vi "AutoDrive.vi"(9 "Initialized":bool) -> (2 "Drive State":T3=enum."Follow Path")   [LabVIEW 2018]
uses:
  driveStateEnum.ctl
  MotionProfile/Path_Decider.ctl
  MotionProfile/StartingPosition.ctl
  AutoDriveStates.ctl
  MotionProfile/AutoOptions.ctl
  Sensors/Limelight/LimelightPipelineMode.ctl
  <userlib>/836-Library/System/TDMS_V2/Support/TDMS_DevRef.ctl
  <userlib>/836-Library/System/TDMS_V2/Support/Logging_Settings.ctl
  <userlib>/836-Library/System/TDMS_V2/Support/Group_FIFO_Config.ctl
  <userlib>/836-Library/System/TDMS_V2/Support/Channel_FIFO_Config.ctl
  HatchPanel/hatchPanelEnum.ctl
  HatchPanel/hatchPanelNotifierCluster.ctl
  Sensors/Limelight/LimelightModeEnum.ctl
  driveShifterEnum.ctl
  MotionProfile/Constants.vi
panel:
  in  "Override Dashboard":bool
  out "Complete Path Valid?":bool
  in  "Starting Position":T1
  in  "Second":T2=enum."5"
  in  "First":T2=enum."7"
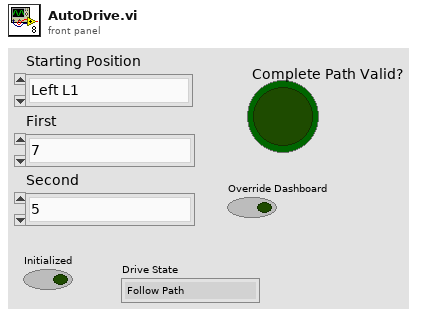
[diagram p1: front panel]
types:
  T1 = typedef "StartingPosition.ctl" = enum16{"Left L1 ", "Middle L1", "Right L1", "Left L2", "Right L2", "Don't Move"}
  T2 = typedef "Path_Decider.ctl" = enum16{"1", "2", "3", "4", "5", "6", "7", "8", "Left_Rocket_Front", "Left_Rocket_Rear", "Right_Rocket_Front", "Right_Rocket_Rear"}
  T3 = typedef "driveStateEnum.ctl" = enum16{"doNothing", "Manuel", "Teleop", "Follow Path (init)", "Follow Path", "Move to Target", "Climb", "Line Align", "Turn to Angle", "Sonar Brake Tele", "Code Drive"}
  T4 = typedef "AutoDriveStates.ctl" = enum16{"1 - MP First leg A (init)", "2 - MP First leg A", "3 - Wait for direction change", "4 - MP First leg B (init)", "5 - MP First leg B", "6 - Wait for shift", "7 - Aproach to score", "8 - Scored", "9 - MP Second leg A (init)", "10 - MP Second leg A", "11 - Wait for direction change", "12 - MP Second leg B (init)", "13 - MP Second leg B", "14 - Wait for shift", "15 - Extend claw", "16 - Aproach to grab", "17 - Grabbed", "18 - MP Third leg A (init)", "19 - MP Third leg A", "20 - Wait for direction change", "21 - MP Third leg B (init)", "22 - MP Third leg B", "23 - Wait to shift", "24 - Aproach to score", "25 - Scored", "26 - Backup 0.3 Seconds", "27 - doNothing"}
  T5 = typedef "AutoOptions.ctl" = cluster{"Starting Position":T1, "First Score Pos":T2, "Second Score Pos":T2}
  T6 = typedef "LimelightPipelineMode.ctl" = enum16{"Closest", "Leftmost", "Rightmost"}
  T7 = typedef "pathLeg.ctl" = cluster{"First Path":string, "Second Path Needed?":bool, "Second Path":string}
  T8 = typedef "WPI_MotorControlDeviceRef.ctl" = cluster{"DeviceStatus":errorcluster, "Type":T9, "PWM":cluster{"PWM Channel":T10, "DeadBand":T11}, "CAN":cluster{"Device Number":u8, "SetOutput VI Ref":variant, "GetOutput VI Ref":variant, "Enable VI Ref":variant, "Disable VI Ref":variant, "Data":variant}, "Invert":bool, "DIO PWM":cluster{"PWM \"Enable\" Channel":T10, "DIOChannel":T12, "PWM Rate":dbl}}
  T9 = typedef "WPI_MotorControlType.ctl" = enum16{"PWM", "CAN", "DIO PWM"}
  T10 = typedef "FPGA_DIOPWMChannel.ctl" = enum8{"PWM 0", "PWM 1", "PWM 2", "PWM 3", "PWM 4", "PWM 5", "PWM 6", "PWM 7", "PWM 8", "PWM 9", "PWM MXP 0", "PWM MXP 1", "PWM MXP 2", "PWM MXP 3", "PWM MXP 4", "PWM MXP 5", "PWM MXP 6", "PWM MXP 7", "PWM MXP 8", "PWM MXP 9", "Invalid"}
  T11 = typedef "WPI_PWMDeadband.ctl" = cluster{"Name":string, "maxPositivePwm":i32, "minPositivePwm":i32, "centerPwm":i32, "maxNegativePwm":i32, "minNegativePwm":i32, "angularRange":u16}
  T12 = typedef "FPGA_DIOChannel.ctl" = enum8{"DIO 0", "DIO 1", "DIO 2", "DIO 3", "DIO 4", "DIO 5", "DIO 6", "DIO 7", "DIO 8", "DIO 9", "DIO MXP 0", "DIO MXP 1", "DIO MXP 2", "DIO MXP 3", "DIO MXP 4", "DIO MXP 5", "DIO MXP 6", "DIO MXP 7", "DIO MXP 8", "DIO MXP 9", "DIO MXP 10", "DIO MXP 11", "DIO MXP 12", "DIO MXP 13", "DIO MXP 14", "DIO MXP 15", "SPI Port CS1", "SPI Port CS2", "SPI Port CS3", "SPI Port MISO", "SPI Port MOSI", "Invalid"}
  T13 = typedef "driveShifterEnum.ctl" = enum16{"Low", "High"}
  T14 = typedef "LimelightModeEnum.ctl" = enum16{"SA - Front", "SA - Rear", "SA - Side by Side", "Vision Processing"}
  T15 = typedef "hatchPanelNotifierCluster.ctl" = cluster{"Hatch Panel State":T16, "Mechanism Motion":bool, "Gathering Claw Motion":bool, "Scoring Claw Motion":bool}
  T16 = typedef "hatchPanelEnum.ctl" = enum16{"do nothing", "Stach Mode", "Climb Mode", "Retracted Closed", "Retracted Open", "Extended Closed", "Extended Open"}
  T17 = typedef "CTRE_PigeonIMU_DeviceRef.ctl" = cluster{"DeviceStatus":errorcluster, "Device Number":u8, "Type":T18, "Device ID":u32, "Handle":u64, "UsageFrame":u32, "Library Path":path}
  T18 = typedef "CTRE_PigeonIMU_ConnectionType.ctl" = u32
  T19 = typedef "TDMS_DevRef.ctl" = cluster{"Name":string, "File Ref":refnum<k34>, "Start Time":timestamp, "Logging Settings":T20, "Group FIFO Config":T21[], "Data To Write":refnum<data-value>, "semaphore":T23, "Ref Time Reset":refnum<k4>}
  T20 = typedef "Logging_Settings.ctl" = cluster{"Data Grab Period":dbl, "File Write Period":dbl, "Max Stored Size":dbl, "Burst Size":dbl}
  T21 = typedef "Group_FIFO_Config.ctl" = cluster{"Group":string, "Channels":T22[], "Channel Names":string[]}
  T22 = typedef "Channel_FIFO_Config.ctl" = cluster{"Channel":string, "FIFO":refnum<k33>}
  T23 = typedef "Semaphore RefNum" = refnum<k1>
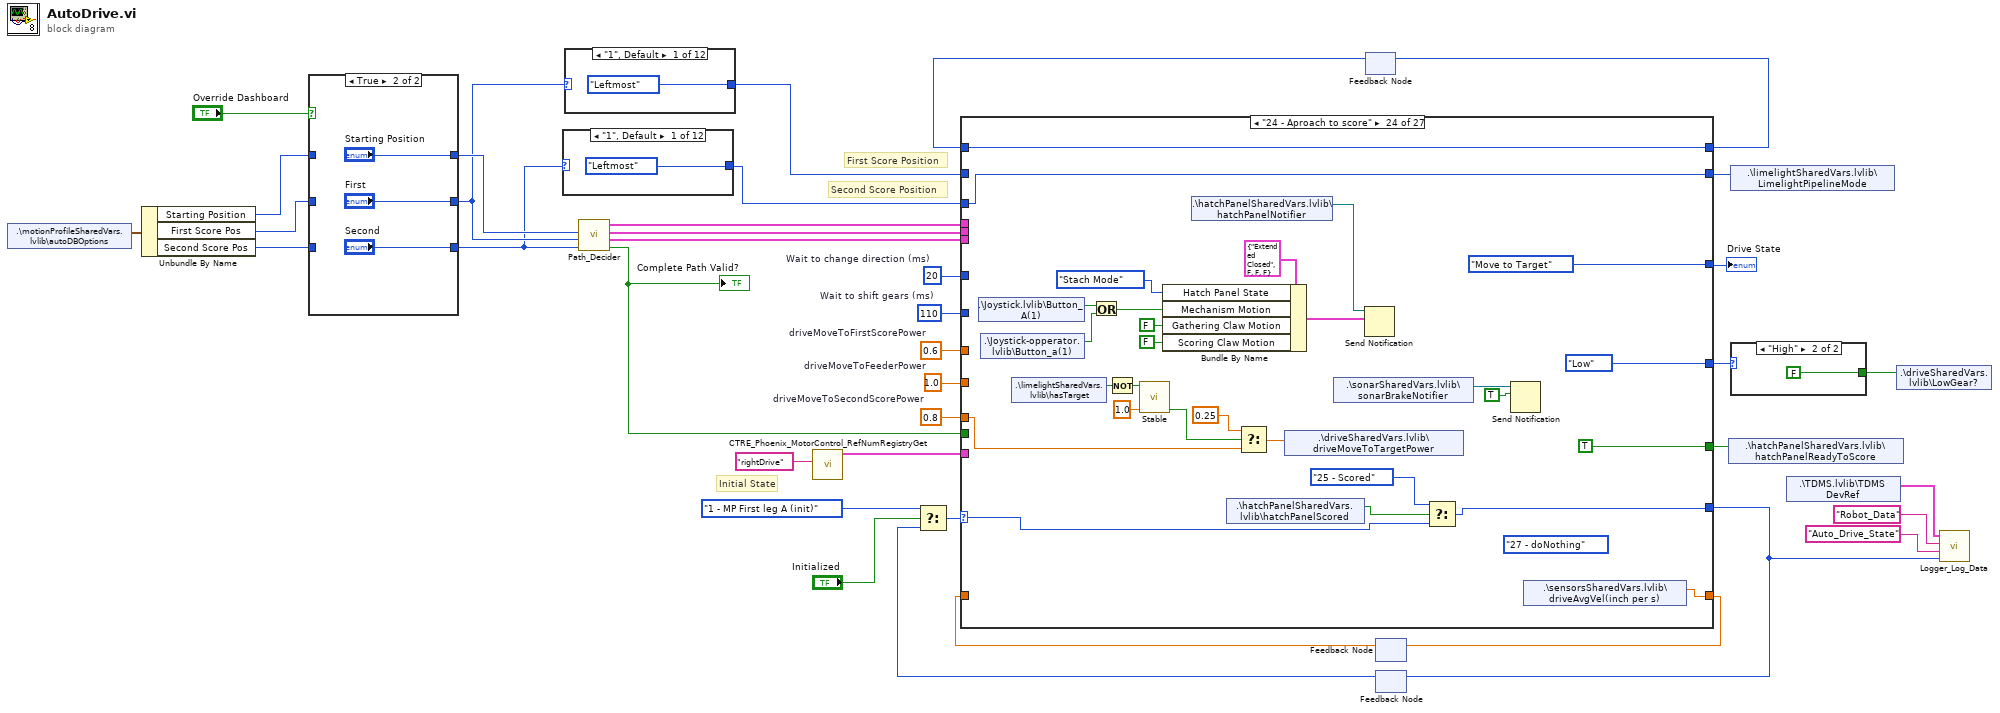
[diagram p0: block diagram]
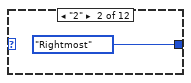
[diagram p2: hidden frame]
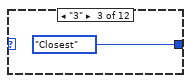
[diagram p3: hidden frame]
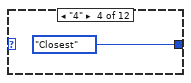
[diagram p4: hidden frame]
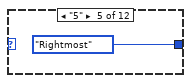
[diagram p5: hidden frame]
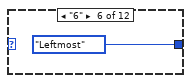
[diagram p6: hidden frame]
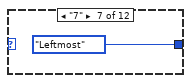
[diagram p7: hidden frame]
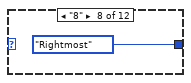
[diagram p8: hidden frame]
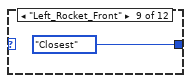
[diagram p9: hidden frame]
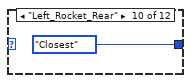
[diagram p10: hidden frame]
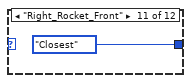
[diagram p11: hidden frame]
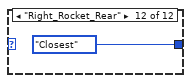
[diagram p12: hidden frame]
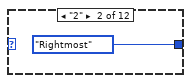
[diagram p13: hidden frame]
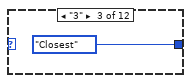
[diagram p14: hidden frame]
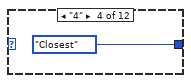
[diagram p15: hidden frame]
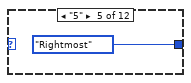
[diagram p16: hidden frame]
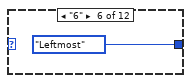
[diagram p17: hidden frame]
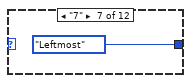
[diagram p18: hidden frame]
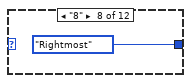
[diagram p19: hidden frame]
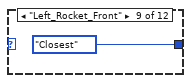
[diagram p20: hidden frame]
diagram:
  w9 = 0.8  # driveMoveToSecondScorePower
  w10 = 1.0  # driveMoveToFeederPower
  w23 = 0.6  # driveMoveToFirstScorePower
  w24 = u32 110  # Wait to shift gears (ms)
  w25 = u32 20  # Wait to change direction (ms)
  # "Second Score Position"
  # "First Score Position"
  # "Initial State"
  n1 = shared-variable ".\\motionProfileSharedVars.lvlib\\autoDBOptions"() -> (w17:T5)  [unwired: 1 in, 1 out]
  n2 = Unbundle By Name(w17) -> ("Starting Position"=w19:T1, "First Score Pos"=w20:T2, "Second Score Pos"=w21:T2)
  n3 = case shown="True" "Override Dashboard" {
    tunnel: [w40 "First"] -> w5
    tunnel: [w41 "Second"] -> w2
    tunnel: [w39 "Starting Position"] -> w6
    tunnel: w21 -> [w41 _]
    tunnel: w20 -> [w40 _]
    tunnel: w19 -> [w39 _]
    frame False {
    }
    frame True {
    }
  }
  n4 = case shown="\"1\", Default" w2 {
    tunnel: [LimelightPipelineMode."Leftmost" ("Enum") LimelightPipelineMode."Rightmost" ("Enum") LimelightPipelineMode."Closest" ("Enum") LimelightPipelineMode."Closest" ("Enum") LimelightPipelineMode."Rightmost" ("Enum") LimelightPipelineMode."Leftmost" ("Enum") LimelightPipelineMode."Leftmost" ("Enum") LimelightPipelineMode."Rightmost" ("Enum") LimelightPipelineMode."Closest" ("Enum") LimelightPipelineMode."Closest" ("Enum") LimelightPipelineMode."Closest" ("Enum") LimelightPipelineMode."Closest" ("Enum")] -> w1
    frame "1", Default {
    }
    frame "2" {
    }
    frame "3" {
    }
    frame "4" {
    }
    frame "5" {
    }
    frame "6" {
    }
    frame "7" {
    }
    frame "8" {
    }
    frame "Left_Rocket_Front" {
    }
    frame "Left_Rocket_Rear" {
    }
    frame "Right_Rocket_Front" {
    }
    frame "Right_Rocket_Rear" {
    }
  }
  n5 = case shown="\"1\", Default" w5 {
    tunnel: [LimelightPipelineMode."Leftmost" ("Enum") LimelightPipelineMode."Rightmost" ("Enum") LimelightPipelineMode."Closest" ("Enum") LimelightPipelineMode."Closest" ("Enum") LimelightPipelineMode."Rightmost" ("Enum") LimelightPipelineMode."Leftmost" ("Enum") LimelightPipelineMode."Leftmost" ("Enum") LimelightPipelineMode."Rightmost" ("Enum") LimelightPipelineMode."Closest" ("Enum") LimelightPipelineMode."Closest" ("Enum") LimelightPipelineMode."Closest" ("Enum") LimelightPipelineMode."Closest" ("Enum")] -> w4
    frame "1", Default {
    }
    frame "2" {
    }
    frame "3" {
    }
    frame "4" {
    }
    frame "5" {
    }
    frame "6" {
    }
    frame "7" {
    }
    frame "8" {
    }
    frame "Left_Rocket_Front" {
    }
    frame "Left_Rocket_Rear" {
    }
    frame "Right_Rocket_Front" {
    }
    frame "Right_Rocket_Rear" {
    }
  }
  n6 = call "Path_Decider.vi"("Second"=w2, "First"=w5, "Starting Position"=w6) -> ("Complete Path Valid?"=w18:bool, "Score Second HP Leg"=w26:T7, "Retrieve Second HP Leg"=w27:T7, "Score First HP Leg"=w28:T7)  [unwired: 4 in]
  "Complete Path Valid?" <- w18
  n7 = call <vilib>:"CTRE_Phoenix_MotorControl_RefNumRegistryGet.vi"("refnum name"="rightDrive") -> ("PhoenixMotorControlDevRef"=w37:T8)  [unwired: 9 in, 1 out]
  n8 = feedback #1() -> (w33:u32)  [unwired: 1 in]
  n9 = feedback #2() -> (w7:dbl)  [unwired: 1 in]
  n10 = feedback #3() -> (w29:T4)  [unwired: 1 in]
  n11 = Select(t=AutoDriveStates."1 - MP First leg A (init)" ("Enum"), s="Initialized", f=w29) -> (s? t:f=w30:T4)
  n12 = case shown="\"24 - Aproach to score\"" w30 {
    selector: w30 -> [_ w122 w139 _ w175 w184 w217 _ _ w272 w293 _ w333 w341 _ w376 _ _ w450 w471 _ w507 w516 w548 _ w576 _]
    tunnel: [w86 w101 w124 AutoDriveStates."5 - MP First leg B" ("Enum") w177 w183 w194 AutoDriveStates."9 - MP Second leg A (init)" ("Enum") AutoDriveStates."10 - MP Second leg A" ("Enum") w271 w278 AutoDriveStates."13 - MP Second leg B" ("Enum") w320 w335 AutoDriveStates."16 - Aproach to grab" ("t") w355 AutoDriveStates."18 - MP Third leg A (init)" ("Enum") AutoDriveStates."19 - MP Third leg A" ("Enum") w449 w456 AutoDriveStates."22 - MP Third leg B" ("Enum") w506 w515 w526 AutoDriveStates."26 - Backup 0.3 Seconds" ("Enum") w575 AutoDriveStates."27 - doNothing" ("Enum")] -> w11
    tunnel: [driveStateEnum."Follow Path (init)" ("Drive State Enum") driveStateEnum."Follow Path" ("Drive State Enum") driveStateEnum."doNothing" ("Drive State Enum") driveStateEnum."Follow Path (init)" ("Drive State Enum") driveStateEnum."Follow Path" ("Drive State Enum") driveStateEnum."doNothing" ("Drive State Enum") driveStateEnum."Move to Target" ("Drive State Enum") driveStateEnum."doNothing" ("Drive State Enum") driveStateEnum."Follow Path (init)" ("Drive State Enum") driveStateEnum."Follow Path" ("Drive State Enum") driveStateEnum."doNothing" ("Drive State Enum") driveStateEnum."Follow Path (init)" ("Drive State Enum") driveStateEnum."Follow Path" ("Drive State Enum") driveStateEnum."doNothing" ("Drive State Enum") driveStateEnum."doNothing" ("Drive State Enum") driveStateEnum."Move to Target" ("Drive State Enum") driveStateEnum."doNothing" ("Drive State Enum") driveStateEnum."Follow Path (init)" ("Drive State Enum") driveStateEnum."Follow Path" ("Drive State Enum") driveStateEnum."doNothing" ("Drive State Enum") driveStateEnum."Follow Path (init)" ("Drive State Enum") driveStateEnum."Follow Path" ("Drive State Enum") driveStateEnum."doNothing" ("Drive State Enum") driveStateEnum."Move to Target" ("Drive State Enum") driveStateEnum."doNothing" ("Drive State Enum") driveStateEnum."Code Drive" ("Drive State Enum") driveStateEnum."doNothing" ("Drive State Enum")] -> w35
    tunnel: w37 -> [_ w121 _ _ w176 _ _ _ _ w273 _ _ w332 _ _ _ _ _ w451 _ _ w508 _ _ _ _ _]
    tunnel: [w73 w109 w130 w148 w167 driveShifterEnum."Low" ("driveShifterPosition") driveShifterEnum."Low" ("driveShifterPosition") driveShifterEnum."Low" ("driveShifterPosition") w242 w261 w284 w302 w322 driveShifterEnum."Low" ("driveShifterPosition") driveShifterEnum."Low" ("driveShifterPosition") driveShifterEnum."Low" ("driveShifterPosition") driveShifterEnum."High" ("driveShifterPosition") w401 w439 w462 w480 w499 driveShifterEnum."Low" ("driveShifterPosition") driveShifterEnum."Low" ("driveShifterPosition") driveShifterEnum."Low" ("driveShifterPosition") driveShifterEnum."Low" ("driveShifterPosition") driveShifterEnum."High" ("driveShifterPosition")] -> w16
    tunnel: [w97 w119 w143 w157 w173 w186 w220 w235 w253 w274 w297 w311 w330 w345 w352 w378 w393 w418 w452 w475 w489 w509 w518 w551 w563 w577 w588] -> w34
    tunnel: w33 -> [w97 _ w143 w157 _ w186 w220 w235 w253 _ w297 w311 _ w345 w352 w378 w393 w418 _ w475 w489 _ w518 w551 _ w577 w588]
    tunnel: [FALSE FALSE FALSE FALSE FALSE FALSE TRUE FALSE FALSE FALSE FALSE FALSE FALSE FALSE TRUE TRUE FALSE FALSE FALSE FALSE FALSE FALSE FALSE TRUE FALSE FALSE FALSE] -> w32
    tunnel: w28 -> [w87 w117 w128 w155 w174 _ _ _ _ _ _ _ _ _ _ _ _ _ _ _ _ _ _ _ _ _ _]
    tunnel: w27 -> [_ _ _ _ _ _ _ _ w249 w270 w282 w309 w328 _ _ _ _ _ _ _ _ _ _ _ _ _ _]
    tunnel: w26 -> [_ _ _ _ _ _ _ _ _ _ _ _ _ _ _ _ _ w416 w445 w460 w487 w505 _ _ _ _ _]
    tunnel: w25 -> [_ _ w137 _ _ _ _ _ _ _ w291 _ _ _ _ _ _ _ _ w469 _ _ _ _ _ _ _]
    tunnel: w24 -> [_ _ _ _ _ w185 _ _ _ _ _ _ _ w338 _ _ _ _ _ _ _ _ w517 _ _ _ _]
    tunnel: w23 -> [_ _ _ _ _ _ _ _ _ _ _ _ _ _ _ _ _ _ _ _ _ _ _ _ _ _ _]
    tunnel: w18 -> [w84 _ _ _ _ _ _ _ _ _ _ _ _ _ _ _ _ _ _ _ _ _ _ _ _ _ _]
    tunnel: w10 -> [_ _ _ _ _ _ _ _ _ _ _ _ _ _ _ w365 _ _ _ _ _ _ _ _ _ _ _]
    tunnel: w9 -> [_ _ _ _ _ _ _ _ _ _ _ _ _ _ _ _ _ _ _ _ _ _ _ w538 _ _ _]
    tunnel: [w70 w102 w127 w146 w161 w182 w204 w231 w240 w255 w281 w300 w315 w337 w349 w364 w389 w399 w433 w459 w478 w493 w514 w537 w562 w571 w586] -> w8
    tunnel: w7 -> [_ _ _ _ _ _ w204 _ _ _ _ _ _ _ _ _ _ _ _ _ _ _ _ _ _ _ w586]
    tunnel: w4 -> [w69 w100 w126 w145 w160 w181 w202 w230 _ _ _ _ _ _ _ _ _ _ _ _ _ _ _ _ _ _ _]
    tunnel: w1 -> [_ _ _ _ _ _ _ _ _ _ _ _ _ _ _ _ _ w398 w432 w458 w477 w492 w513 w536 w561 w570 w585]
    tunnel: [w69 w100 w126 w145 w160 w181 w202 w230 LimelightPipelineMode."Closest" ("Enum") LimelightPipelineMode."Closest" ("Enum") LimelightPipelineMode."Closest" ("Enum") LimelightPipelineMode."Closest" ("Enum") LimelightPipelineMode."Closest" ("Enum") LimelightPipelineMode."Closest" ("Enum") LimelightPipelineMode."Closest" ("Enum") LimelightPipelineMode."Closest" ("Enum") LimelightPipelineMode."Closest" ("Enum") w398 w432 w458 w477 w492 w513 w536 w561 w570 w585] -> w3
    frame "1 - MP First leg A (init)", Default {
      n13 = shared-variable ".\\limelightSharedVars.lvlib\\limelightModeNotifier"() -> (w82:refnum<notifier>)  [unwired: 1 in, 1 out]
      n14 = shared-variable ".\\sonarSharedVars.lvlib\\sonarBrakeNotifier"() -> (w72:refnum<notifier>)  [unwired: 1 in, 1 out]
      n15 = Unbundle By Name(w87) -> ("First Path"=w74:string)
      n16 = call <vilib>:"CTRE_PigeonIMU_RefNumRegistryGet.vi"("refnum name"="driveIMU") -> ("PigeonIMUDevRef"=w88:T17)  [unwired: 9 in, 1 out]
      n17 = call "ZeroPigeon.vi"("Pigeon"=w88) -> ()  [unwired: 8 in, 1 out]
      n18 = shared-variable ".\\motionProfileSharedVars.lvlib\\motionProfilePathName"(w74) -> ()  [unwired: 1 in, 1 out]
      n19 = Send Notification(notification=LimelightModeEnum."Vision Processing", notifier=w82) -> ()  [unwired: 1 in, 2 out]
      n20 = Send Notification(notification=FALSE, notifier=w72) -> ()  [unwired: 1 in, 2 out]
      n21 = Bundle By Name(cluster=T15 {"Hatch Panel State"=enum."Extended Closed", "Mechanism Motion"=FALSE, "Gathering Claw Motion"=FALSE, "Scoring Claw Motion"=FALSE} ("notification"), "Hatch Panel State"=hatchPanelEnum."Stach Mode", "Mechanism Motion"=FALSE, "Gathering Claw Motion"=FALSE, "Scoring Claw Motion"=FALSE) -> (w94:T15)
      n22 = String Subset(string=w74, length (rest)=4 ("length (rest)")) -> (substring=w79:string)  [unwired: 1 in]
      n23 = shared-variable ".\\hatchPanelSharedVars.lvlib\\hatchPanelNotifier"() -> (w95:refnum<notifier>)  [unwired: 1 in, 1 out]
      n24 = Equal?(x="low_", y=w79) -> (x = y?=w75:bool)
      n25 = Send Notification(notification=w94, notifier=w95) -> ()  [unwired: 1 in, 2 out]
      n26 = shared-variable ".\\sensorsSharedVars.lvlib\\driveAvgVel(inch per s)"() -> (w70:dbl)  [unwired: 1 in, 1 out]
      n27 = Select(t=driveShifterEnum."Low" ("driveShifterPosition"), s=w75, f=driveShifterEnum."High" ("driveShifterPosition")) -> (s? t:f=w73:T13)
      n28 = Select(t=AutoDriveStates."2 - MP First leg A" ("Enum"), s=w84, f=AutoDriveStates."27 - doNothing" ("Enum")) -> (s? t:f=w86:T4)
    }
    frame "2 - MP First leg A" {
      n29 = call <vilib>:"CTRE_Phoenix_MotorControl_IsMotionProfileFinished.vi"("PhoenixMotorControlDevRef"=w121) -> ("Is Motion Profile Finished?"=w120:bool)  [unwired: 8 in, 2 out]
      n30 = Unbundle By Name(w117) -> ("First Path"=w110:string, "Second Path Needed?"=w114:bool)
      n31 = shared-variable ".\\motionProfileSharedVars.lvlib\\motionProfilePathName"(w110) -> ()  [unwired: 1 in, 1 out]
      n32 = String Subset(string=w110, length (rest)=4 ("length (rest)")) -> (substring=w112:string)  [unwired: 1 in]
      n33 = Equal?(x="low_", y=w112) -> (x = y?=w105:bool)
      n34 = shared-variable ".\\sensorsSharedVars.lvlib\\driveAvgVel(inch per s)"() -> (w102:dbl)  [unwired: 1 in, 1 out]
      n35 = Select(t=AutoDriveStates."7 - Aproach to score", s=w105, f=AutoDriveStates."6 - Wait for shift" ("t")) -> (s? t:f=w106:T4)
      n36 = Select(t=AutoDriveStates."3 - Wait for direction change", s=w114, f=w106) -> (s? t:f=w116:T4)
      n37 = Select(t=w116, s=w120, f=w122) -> (s? t:f=w101:T4)
      n38 = Tick Count (ms)() -> (millisecond timer value=w119:u32)
      n39 = Select(t=driveShifterEnum."Low" ("driveShifterPosition"), s=w105, f=driveShifterEnum."High" ("driveShifterPosition")) -> (s? t:f=w109:T13)
    }
    frame "3 - Wait for direction change" {
      n40 = Add(x=w143, y=w137) -> (x+y=w141:u32)
      n41 = Unbundle By Name(w128) -> ("Second Path"=w129:string)
      n42 = Tick Count (ms)() -> (millisecond timer value=w142:u32)
      n43 = Greater Or Equal?(x=w142, y=w141) -> (x >= y?=w140:bool)
      n44 = String Subset(string=w129, length (rest)=4 ("length (rest)")) -> (substring=w135:string)  [unwired: 1 in]
      n45 = Equal?(x="low_", y=w135) -> (x = y?=w131:bool)
      n46 = shared-variable ".\\sensorsSharedVars.lvlib\\driveAvgVel(inch per s)"() -> (w127:dbl)  [unwired: 1 in, 1 out]
      n47 = Select(t=AutoDriveStates."4 - MP First leg B (init)", s=w140, f=w139) -> (s? t:f=w124:T4)
      n48 = Select(t=driveShifterEnum."Low" ("driveShifterPosition"), s=w131, f=driveShifterEnum."High" ("driveShifterPosition")) -> (s? t:f=w130:T13)
    }
    frame "4 - MP First leg B (init)" {
      n49 = Unbundle By Name(w155) -> ("Second Path"=w147:string)
      n50 = shared-variable ".\\motionProfileSharedVars.lvlib\\motionProfilePathName"(w147) -> ()  [unwired: 1 in, 1 out]
      n51 = String Subset(string=w147, length (rest)=4 ("length (rest)")) -> (substring=w153:string)  [unwired: 1 in]
      n52 = Equal?(x="low_", y=w153) -> (x = y?=w149:bool)
      n53 = shared-variable ".\\sensorsSharedVars.lvlib\\driveAvgVel(inch per s)"() -> (w146:dbl)  [unwired: 1 in, 1 out]
      n54 = Select(t=driveShifterEnum."Low" ("driveShifterPosition"), s=w149, f=driveShifterEnum."High" ("driveShifterPosition")) -> (s? t:f=w148:T13)
    }
    frame "5 - MP First leg B" {
      n55 = Unbundle By Name(w174) -> ("Second Path"=w166:string)
      n56 = call <vilib>:"CTRE_Phoenix_MotorControl_IsMotionProfileFinished.vi"("PhoenixMotorControlDevRef"=w176) -> ("Is Motion Profile Finished?"=w178:bool)  [unwired: 8 in, 2 out]
      n57 = shared-variable ".\\motionProfileSharedVars.lvlib\\motionProfilePathName"(w166) -> ()  [unwired: 1 in, 1 out]
      n58 = String Subset(string=w166, length (rest)=4 ("length (rest)")) -> (substring=w171:string)  [unwired: 1 in]
      n59 = Equal?(x="low_", y=w171) -> (x = y?=w162:bool)
      n60 = Select(t=AutoDriveStates."7 - Aproach to score" ("Enum"), s=w162, f=AutoDriveStates."6 - Wait for shift" ("Enum")) -> (s? t:f=w164:T4)
      n61 = shared-variable ".\\sensorsSharedVars.lvlib\\driveAvgVel(inch per s)"() -> (w161:dbl)  [unwired: 1 in, 1 out]
      n62 = Select(t=w164, s=w178, f=w175) -> (s? t:f=w177:T4)
      n63 = Tick Count (ms)() -> (millisecond timer value=w173:u32)
      n64 = Select(t=driveShifterEnum."Low" ("driveShifterPosition"), s=w162, f=driveShifterEnum."High" ("driveShifterPosition")) -> (s? t:f=w167:T13)
    }
    frame "6 - Wait for shift" {
      n65 = Add(x=w186, y=w185) -> (x+y=w189:u32)
      n66 = Tick Count (ms)() -> (millisecond timer value=w190:u32)
      n67 = Greater Or Equal?(x=w190, y=w189) -> (x >= y?=w188:bool)
      n68 = shared-variable ".\\sensorsSharedVars.lvlib\\driveAvgVel(inch per s)"() -> (w182:dbl)  [unwired: 1 in, 1 out]
      n69 = Select(t=AutoDriveStates."7 - Aproach to score", s=w188, f=w184) -> (s? t:f=w183:T4)
    }
    frame "7 - Aproach to score" {
      (unwired) AutoDriveStates."27 - doNothing" ("t")
      w207 = 100.0  # MaxLowGearSpeed (in/s)
      # "8.34457 ft/s Max Low Gear Speed"
      n70 = shared-variable ".\\limelightSharedVars.lvlib\\hasTarget"() -> (w213:bool)  [unwired: 1 in, 1 out]
      n71 = Not(x=w213) -> (.not. x?=w212:bool)
      n72 = Bundle By Name(cluster=T15 {"Hatch Panel State"=enum."Extended Closed", "Mechanism Motion"=FALSE, "Gathering Claw Motion"=FALSE, "Scoring Claw Motion"=FALSE} ("notification"), "Hatch Panel State"=hatchPanelEnum."Stach Mode", "Mechanism Motion"=TRUE, "Gathering Claw Motion"=FALSE, "Scoring Claw Motion"=FALSE) -> (w200:T15)
      n73 = Divide(x=w204, y=w207) -> (x/y=w206:dbl)
      n74 = shared-variable ".\\hatchPanelSharedVars.lvlib\\hatchPanelNotifier"() -> (w201:refnum<notifier>)  [unwired: 1 in, 1 out]
      n75 = call <userlib>:"Stable.vi"("Eval Period (sec)"=0.5, "Signal Input"=w212) -> ("Stable"=w210:bool)  [unwired: 9 in]
      n76 = Divide(x=w206, y=0.64) -> (x/y=w203:dbl)
      n77 = Select(t=0.25, s=w210, f=w203) -> (s? t:f=w208:dbl)
      n78 = shared-variable ".\\driveSharedVars.lvlib\\driveMoveToTargetPower"(w208) -> ()  [unwired: 1 in, 1 out]
      n79 = Send Notification(notification=w200, notifier=w201) -> ()  [unwired: 1 in, 2 out]
      n80 = shared-variable ".\\hatchPanelSharedVars.lvlib\\hatchPanelScored"() -> (w218:bool)  [unwired: 1 in, 1 out]
      n81 = shared-variable ".\\sonarSharedVars.lvlib\\sonarBrakeNotifier"() -> (w216:refnum<notifier>)  [unwired: 1 in, 1 out]
      n82 = Select(t=AutoDriveStates."8 - Scored", s=w218, f=w217) -> (s? t:f=w194:T4)
      n83 = Send Notification(notification=TRUE, notifier=w216) -> ()  [unwired: 1 in, 2 out]
    }
    frame "8 - Scored" {
      n84 = Bundle By Name(cluster=T15 {"Hatch Panel State"=enum."Extended Closed", "Mechanism Motion"=FALSE, "Gathering Claw Motion"=FALSE, "Scoring Claw Motion"=FALSE} ("notification"), "Hatch Panel State"=hatchPanelEnum."Stach Mode", "Mechanism Motion"=FALSE, "Gathering Claw Motion"=FALSE, "Scoring Claw Motion"=FALSE) -> (w228:T15)
      n85 = shared-variable ".\\hatchPanelSharedVars.lvlib\\hatchPanelNotifier"() -> (w229:refnum<notifier>)  [unwired: 1 in, 1 out]
      n86 = shared-variable ".\\sonarSharedVars.lvlib\\sonarBrakeNotifier"() -> (w234:refnum<notifier>)  [unwired: 1 in, 1 out]
      n87 = Send Notification(notification=w228, notifier=w229) -> ()  [unwired: 1 in, 2 out]
      n88 = Send Notification(notification=FALSE, notifier=w234) -> ()  [unwired: 1 in, 2 out]
      n89 = shared-variable ".\\sensorsSharedVars.lvlib\\driveAvgVel(inch per s)"() -> (w231:dbl)  [unwired: 1 in, 1 out]
    }
    frame "9 - MP Second leg A (init)" {
      n90 = Unbundle By Name(w249) -> ("First Path"=w241:string)
      n91 = shared-variable ".\\motionProfileSharedVars.lvlib\\motionProfilePathName"(w241) -> ()  [unwired: 1 in, 1 out]
      n92 = String Subset(string=w241, length (rest)=4 ("length (rest)")) -> (substring=w247:string)  [unwired: 1 in]
      n93 = Equal?(x="low_", y=w247) -> (x = y?=w243:bool)
      n94 = shared-variable ".\\sensorsSharedVars.lvlib\\driveAvgVel(inch per s)"() -> (w240:dbl)  [unwired: 1 in, 1 out]
      n95 = Select(t=driveShifterEnum."Low" ("driveShifterPosition"), s=w243, f=driveShifterEnum."High" ("driveShifterPosition")) -> (s? t:f=w242:T13)
    }
    frame "10 - MP Second leg A" {
      n96 = call <vilib>:"CTRE_Phoenix_MotorControl_IsMotionProfileFinished.vi"("PhoenixMotorControlDevRef"=w273) -> ("Is Motion Profile Finished?"=w275:bool)  [unwired: 8 in, 2 out]
      n97 = Unbundle By Name(w270) -> ("First Path"=w260:string, "Second Path Needed?"=w267:bool)
      n98 = shared-variable ".\\motionProfileSharedVars.lvlib\\motionProfilePathName"(w260) -> ()  [unwired: 1 in, 1 out]
      n99 = String Subset(string=w260, length (rest)=4 ("length (rest)")) -> (substring=w265:string)  [unwired: 1 in]
      n100 = Equal?(x="low_", y=w265) -> (x = y?=w258:bool)
      n101 = Select(t=AutoDriveStates."16 - Aproach to grab", s=w258, f=AutoDriveStates."14 - Wait for shift" ("t")) -> (s? t:f=w257:T4)
      n102 = shared-variable ".\\sensorsSharedVars.lvlib\\driveAvgVel(inch per s)"() -> (w255:dbl)  [unwired: 1 in, 1 out]
      n103 = Select(t=AutoDriveStates."11 - Wait for direction change", s=w267, f=w257) -> (s? t:f=w269:T4)
      n104 = Select(t=w269, s=w275, f=w272) -> (s? t:f=w271:T4)
      n105 = Tick Count (ms)() -> (millisecond timer value=w274:u32)
      n106 = Select(t=driveShifterEnum."Low" ("driveShifterPosition"), s=w258, f=driveShifterEnum."High" ("driveShifterPosition")) -> (s? t:f=w261:T13)
    }
    frame "11 - Wait for direction change" {
      (unwired) AutoDriveStates."27 - doNothing" ("t")
      n107 = Add(x=w297, y=w291) -> (x+y=w295:u32)
      n108 = Unbundle By Name(w282) -> ("Second Path"=w283:string)
      n109 = Tick Count (ms)() -> (millisecond timer value=w296:u32)
      n110 = Greater Or Equal?(x=w296, y=w295) -> (x >= y?=w294:bool)
      n111 = String Subset(string=w283, length (rest)=4 ("length (rest)")) -> (substring=w289:string)  [unwired: 1 in]
      n112 = Equal?(x="low_", y=w289) -> (x = y?=w285:bool)
      n113 = shared-variable ".\\sensorsSharedVars.lvlib\\driveAvgVel(inch per s)"() -> (w281:dbl)  [unwired: 1 in, 1 out]
      n114 = Select(t=AutoDriveStates."12 - MP Second leg B (init)", s=w294, f=w293) -> (s? t:f=w278:T4)
      n115 = Select(t=driveShifterEnum."Low" ("driveShifterPosition"), s=w285, f=driveShifterEnum."High" ("driveShifterPosition")) -> (s? t:f=w284:T13)
    }
    frame "12 - MP Second leg B (init)" {
      n116 = Unbundle By Name(w309) -> ("Second Path"=w301:string)
      n117 = shared-variable ".\\motionProfileSharedVars.lvlib\\motionProfilePathName"(w301) -> ()  [unwired: 1 in, 1 out]
      n118 = String Subset(string=w301, length (rest)=4 ("length (rest)")) -> (substring=w307:string)  [unwired: 1 in]
      n119 = Equal?(x="low_", y=w307) -> (x = y?=w303:bool)
      n120 = shared-variable ".\\sensorsSharedVars.lvlib\\driveAvgVel(inch per s)"() -> (w300:dbl)  [unwired: 1 in, 1 out]
      n121 = Select(t=driveShifterEnum."Low" ("driveShifterPosition"), s=w303, f=driveShifterEnum."High" ("driveShifterPosition")) -> (s? t:f=w302:T13)
    }
    frame "13 - MP Second leg B" {
      n122 = call <vilib>:"CTRE_Phoenix_MotorControl_IsMotionProfileFinished.vi"("PhoenixMotorControlDevRef"=w332) -> ("Is Motion Profile Finished?"=w331:bool)  [unwired: 8 in, 2 out]
      n123 = Unbundle By Name(w328) -> ("Second Path"=w321:string)
      n124 = shared-variable ".\\motionProfileSharedVars.lvlib\\motionProfilePathName"(w321) -> ()  [unwired: 1 in, 1 out]
      n125 = String Subset(string=w321, length (rest)=4 ("length (rest)")) -> (substring=w326:string)  [unwired: 1 in]
      n126 = Equal?(x="low_", y=w326) -> (x = y?=w316:bool)
      n127 = Select(t=AutoDriveStates."16 - Aproach to grab", s=w316, f=AutoDriveStates."14 - Wait for shift" ("t")) -> (s? t:f=w319:T4)
      n128 = shared-variable ".\\sensorsSharedVars.lvlib\\driveAvgVel(inch per s)"() -> (w315:dbl)  [unwired: 1 in, 1 out]
      n129 = Select(t=w319, s=w331, f=w333) -> (s? t:f=w320:T4)
      n130 = Select(t=driveShifterEnum."Low" ("driveShifterPosition"), s=w316, f=driveShifterEnum."High" ("driveShifterPosition")) -> (s? t:f=w322:T13)
      n131 = Tick Count (ms)() -> (millisecond timer value=w330:u32)
    }
    frame "14 - Wait for shift" {
      n132 = Add(x=w345, y=w338) -> (x+y=w343:u32)
      n133 = Tick Count (ms)() -> (millisecond timer value=w344:u32)
      n134 = Greater Or Equal?(x=w344, y=w343) -> (x >= y?=w342:bool)
      n135 = shared-variable ".\\sensorsSharedVars.lvlib\\driveAvgVel(inch per s)"() -> (w337:dbl)  [unwired: 1 in, 1 out]
      n136 = Select(t=AutoDriveStates."16 - Aproach to grab", s=w342, f=w341) -> (s? t:f=w335:T4)
    }
    frame "15 - Extend claw" {
      n137 = shared-variable ".\\sensorsSharedVars.lvlib\\driveAvgVel(inch per s)"() -> (w349:dbl)  [unwired: 1 in, 1 out]
    }
    frame "16 - Aproach to grab" {
      (unwired) AutoDriveStates."27 - doNothing" ("t")
      n138 = shared-variable ".\\limelightSharedVars.lvlib\\hasTarget"() -> (w371:bool)  [unwired: 1 in, 1 out]
      n139 = shared-variable ".\\hatchPanelSharedVars.lvlib\\Hatch_Claws_Close?"() -> (w372:bool)  [unwired: 1 in, 1 out]
      n140 = Not(x=w371) -> (.not. x?=w370:bool)
      n141 = Bundle By Name(cluster=T15 {"Hatch Panel State"=enum."Extended Closed", "Mechanism Motion"=FALSE, "Gathering Claw Motion"=FALSE, "Scoring Claw Motion"=FALSE} ("notification"), "Hatch Panel State"=hatchPanelEnum."Stach Mode", "Mechanism Motion"=TRUE, "Gathering Claw Motion"=FALSE, "Scoring Claw Motion"=FALSE) -> (w361:T15)
      n142 = call <userlib>:"Stable.vi"("Eval Period (sec)"=1.0, "Signal Input"=w370) -> ("Stable"=w368:bool)  [unwired: 9 in]
      n143 = shared-variable ".\\hatchPanelSharedVars.lvlib\\hatchPanelNotifier"() -> (w362:refnum<notifier>)  [unwired: 1 in, 1 out]
      n144 = Select(t=0.25, s=w368, f=w365) -> (s? t:f=w366:dbl)
      n145 = shared-variable ".\\driveSharedVars.lvlib\\driveMoveToTargetPower"(w366) -> ()  [unwired: 1 in, 1 out]
      n146 = Send Notification(notification=w361, notifier=w362) -> ()  [unwired: 1 in, 2 out]
      n147 = shared-variable ".\\sonarSharedVars.lvlib\\sonarBrakeNotifier"() -> (w375:refnum<notifier>)  [unwired: 1 in, 1 out]
      n148 = Select(t=AutoDriveStates."17 - Grabbed", s=w372, f=w376) -> (s? t:f=w355:T4)
      n149 = Send Notification(notification=TRUE, notifier=w375) -> ()  [unwired: 1 in, 2 out]
      n150 = shared-variable ".\\sensorsSharedVars.lvlib\\driveAvgVel(inch per s)"() -> (w364:dbl)  [unwired: 1 in, 1 out]
    }
    frame "17 - Grabbed" {
      n151 = Bundle By Name(cluster=T15 {"Hatch Panel State"=enum."Extended Closed", "Mechanism Motion"=FALSE, "Gathering Claw Motion"=FALSE, "Scoring Claw Motion"=FALSE} ("notification"), "Hatch Panel State"=hatchPanelEnum."Stach Mode", "Mechanism Motion"=FALSE, "Gathering Claw Motion"=FALSE, "Scoring Claw Motion"=FALSE) -> (w386:T15)
      n152 = shared-variable ".\\hatchPanelSharedVars.lvlib\\hatchPanelNotifier"() -> (w387:refnum<notifier>)  [unwired: 1 in, 1 out]
      n153 = shared-variable ".\\sonarSharedVars.lvlib\\sonarBrakeNotifier"() -> (w392:refnum<notifier>)  [unwired: 1 in, 1 out]
      n154 = Send Notification(notification=w386, notifier=w387) -> ()  [unwired: 1 in, 2 out]
      n155 = shared-variable ".\\sensorsSharedVars.lvlib\\driveAvgVel(inch per s)"() -> (w389:dbl)  [unwired: 1 in, 1 out]
      n156 = Send Notification(notification=FALSE, notifier=w392) -> ()  [unwired: 1 in, 2 out]
    }
    frame "18 - MP Third leg A (init)" {
      w409 = 360.0 ("y")
      w412 = -160.0 ("y")
      # "Code to fix bounding\nangle issues"
      n157 = shared-variable ".\\sensorsSharedVars.lvlib\\driveIMUYawPitchRoll"() -> (w415:cluster{"Yaw":dbl, "Pitch":dbl, "Roll":dbl})  [unwired: 1 in, 1 out]
      n158 = Unbundle By Name(w416) -> ("First Path"=w400:string)
      n159 = shared-variable ".\\motionProfileSharedVars.lvlib\\motionProfilePathName"(w400) -> ()  [unwired: 1 in, 1 out]
      n160 = Unbundle By Name(w415) -> ("Yaw"=w413:dbl)
      n161 = Negate(x=w412) -> (-x=w414:dbl)
      n162 = String Subset(string=w400, length (rest)=4 ("length (rest)")) -> (substring=w406:string)  [unwired: 1 in]
      n163 = Less Or Equal?(x=w413, y=w412) -> (x <= y?=w411:bool)
      n164 = In Range and Coerce(upper limit=w414, x=w413, lower limit=w412) -> (In Range?=w397:bool)  [unwired: 1 out]
      n165 = Equal?(x="low_", y=w406) -> (x = y?=w402:bool)
      n166 = Negate(x=w409) -> (-x=w410:dbl)
      n167 = Select(t=w409, s=w411, f=w410) -> (s? t:f=w408:dbl)
      n168 = case shown="False" w397 {
        tunnel: w413 -> [w431 _]
        tunnel: w408 -> [w422 _]
        frame False {
          n169 = global read "Constants.vi" "Timeout Ms"() -> (w423:i32)
          n170 = Add(x=w431, y=w422) -> (x+y=w421:dbl)
          n171 = call <vilib>:"CTRE_PigeonIMU_RefNumRegistryGet.vi"("refnum name"="driveIMU") -> ("error out"=w429:errorcluster, "PigeonIMUDevRef"=w428:T17)  [unwired: 9 in]
          n172 = call <vilib>:"CTRE_PigeonIMU_SetYaw.vi"("timeoutMs"=w423, "error in (no error)"=w429, "Value"=w421, "PigeonIMUDevRef"=w428) -> ("error out"=w425:errorcluster, "PigeonIMUDevRef"=w427:T17)  [unwired: 6 in]
          n173 = call <vilib>:"CTRE_PigeonIMU_SetAccumZAngle.vi"("timeoutMs"=w423, "error in (no error)"=w425, "Angle (Deg)"=w421, "PigeonIMUDevRef"=w427) -> ("error out"=w424:errorcluster, "PigeonIMUDevRef"=w426:T17)  [unwired: 6 in]
          n174 = call <vilib>:"CTRE_PigeonIMU_SetFusedHeading.vi"("timeoutMs"=w423, "error in (no error)"=w424, "Value"=w421, "PigeonIMUDevRef 2"=w426) -> ()  [unwired: 6 in, 2 out]
        }
        frame True {
        }
      }
      n175 = shared-variable ".\\sensorsSharedVars.lvlib\\driveAvgVel(inch per s)"() -> (w399:dbl)  [unwired: 1 in, 1 out]
      n176 = Select(t=driveShifterEnum."Low" ("driveShifterPosition"), s=w402, f=driveShifterEnum."High" ("driveShifterPosition")) -> (s? t:f=w401:T13)
    }
    frame "19 - MP Third leg A" {
      n177 = call <vilib>:"CTRE_Phoenix_MotorControl_IsMotionProfileFinished.vi"("PhoenixMotorControlDevRef"=w451) -> ("Is Motion Profile Finished?"=w453:bool)  [unwired: 8 in, 2 out]
      n178 = Unbundle By Name(w445) -> ("First Path"=w438:string, "Second Path Needed?"=w446:bool)
      n179 = shared-variable ".\\motionProfileSharedVars.lvlib\\motionProfilePathName"(w438) -> ()  [unwired: 1 in, 1 out]
      n180 = String Subset(string=w438, length (rest)=4 ("length (rest)")) -> (substring=w443:string)  [unwired: 1 in]
      n181 = Equal?(x="low_", y=w443) -> (x = y?=w435:bool)
      n182 = Select(t=AutoDriveStates."24 - Aproach to score", s=w435, f=AutoDriveStates."23 - Wait to shift" ("t")) -> (s? t:f=w436:T4)
      n183 = shared-variable ".\\sensorsSharedVars.lvlib\\driveAvgVel(inch per s)"() -> (w433:dbl)  [unwired: 1 in, 1 out]
      n184 = Select(t=AutoDriveStates."20 - Wait for direction change", s=w446, f=w436) -> (s? t:f=w448:T4)
      n185 = Select(t=w448, s=w453, f=w450) -> (s? t:f=w449:T4)
      n186 = Select(t=driveShifterEnum."Low" ("driveShifterPosition"), s=w435, f=driveShifterEnum."High" ("driveShifterPosition")) -> (s? t:f=w439:T13)
      n187 = Tick Count (ms)() -> (millisecond timer value=w452:u32)
    }
    frame "20 - Wait for direction change" {
      n188 = Add(x=w475, y=w469) -> (x+y=w473:u32)
      n189 = Unbundle By Name(w460) -> ("Second Path"=w461:string)
      n190 = Tick Count (ms)() -> (millisecond timer value=w474:u32)
      n191 = Greater Or Equal?(x=w474, y=w473) -> (x >= y?=w472:bool)
      n192 = String Subset(string=w461, length (rest)=4 ("length (rest)")) -> (substring=w467:string)  [unwired: 1 in]
      n193 = Equal?(x="low_", y=w467) -> (x = y?=w463:bool)
      n194 = shared-variable ".\\sensorsSharedVars.lvlib\\driveAvgVel(inch per s)"() -> (w459:dbl)  [unwired: 1 in, 1 out]
      n195 = Select(t=AutoDriveStates."21 - MP Third leg B (init)", s=w472, f=w471) -> (s? t:f=w456:T4)
      n196 = Select(t=driveShifterEnum."Low" ("driveShifterPosition"), s=w463, f=driveShifterEnum."High" ("driveShifterPosition")) -> (s? t:f=w462:T13)
    }
    frame "21 - MP Third leg B (init)" {
      n197 = Unbundle By Name(w487) -> ("Second Path"=w479:string)
      n198 = shared-variable ".\\motionProfileSharedVars.lvlib\\motionProfilePathName"(w479) -> ()  [unwired: 1 in, 1 out]
      n199 = String Subset(string=w479, length (rest)=4 ("length (rest)")) -> (substring=w485:string)  [unwired: 1 in]
      n200 = Equal?(x="low_", y=w485) -> (x = y?=w481:bool)
      n201 = shared-variable ".\\sensorsSharedVars.lvlib\\driveAvgVel(inch per s)"() -> (w478:dbl)  [unwired: 1 in, 1 out]
      n202 = Select(t=driveShifterEnum."Low" ("driveShifterPosition"), s=w481, f=driveShifterEnum."High" ("driveShifterPosition")) -> (s? t:f=w480:T13)
    }
    frame "22 - MP Third leg B" {
      n203 = call <vilib>:"CTRE_Phoenix_MotorControl_IsMotionProfileFinished.vi"("PhoenixMotorControlDevRef"=w508) -> ("Is Motion Profile Finished?"=w510:bool)  [unwired: 8 in, 2 out]
      n204 = Unbundle By Name(w505) -> ("Second Path"=w498:string)
      n205 = shared-variable ".\\motionProfileSharedVars.lvlib\\motionProfilePathName"(w498) -> ()  [unwired: 1 in, 1 out]
      n206 = String Subset(string=w498, length (rest)=4 ("length (rest)")) -> (substring=w503:string)  [unwired: 1 in]
      n207 = Equal?(x="low_", y=w503) -> (x = y?=w494:bool)
      n208 = shared-variable ".\\sensorsSharedVars.lvlib\\driveAvgVel(inch per s)"() -> (w493:dbl)  [unwired: 1 in, 1 out]
      n209 = Select(t=AutoDriveStates."24 - Aproach to score", s=w494, f=AutoDriveStates."23 - Wait to shift" ("t")) -> (s? t:f=w497:T4)
      n210 = Select(t=w497, s=w510, f=w507) -> (s? t:f=w506:T4)
      n211 = Tick Count (ms)() -> (millisecond timer value=w509:u32)
      n212 = Select(t=driveShifterEnum."Low" ("driveShifterPosition"), s=w494, f=driveShifterEnum."High" ("driveShifterPosition")) -> (s? t:f=w499:T13)
    }
    frame "23 - Wait to shift" {
      n213 = Add(x=w518, y=w517) -> (x+y=w521:u32)
      n214 = Tick Count (ms)() -> (millisecond timer value=w522:u32)
      n215 = Greater Or Equal?(x=w522, y=w521) -> (x >= y?=w520:bool)
      n216 = shared-variable ".\\sensorsSharedVars.lvlib\\driveAvgVel(inch per s)"() -> (w514:dbl)  [unwired: 1 in, 1 out]
      n217 = Select(t=AutoDriveStates."24 - Aproach to score", s=w520, f=w516) -> (s? t:f=w515:T4)
    }
    frame "24 - Aproach to score" {
      (unwired) AutoDriveStates."27 - doNothing" ("t")
      n218 = shared-variable ".\\Joystick.lvlib\\Button_A(1)"() -> (w529:bool)  [unwired: 1 in, 1 out]
      n219 = shared-variable ".\\Joystick-opperator.lvlib\\Button_a(1)"() -> (w528:bool)  [unwired: 1 in, 1 out]
      n220 = shared-variable ".\\limelightSharedVars.lvlib\\hasTarget"() -> (w544:bool)  [unwired: 1 in, 1 out]
      n221 = Or(x=w529, y=w528) -> (x .or. y?=w527:bool)
      n222 = Not(x=w544) -> (.not. x?=w543:bool)
      n223 = call <userlib>:"Stable.vi"("Eval Period (sec)"=1.0, "Signal Input"=w543) -> ("Stable"=w541:bool)  [unwired: 9 in]
      n224 = Bundle By Name(cluster=T15 {"Hatch Panel State"=enum."Extended Closed", "Mechanism Motion"=FALSE, "Gathering Claw Motion"=FALSE, "Scoring Claw Motion"=FALSE} ("notification"), "Hatch Panel State"=hatchPanelEnum."Stach Mode", "Mechanism Motion"=w527, "Gathering Claw Motion"=FALSE, "Scoring Claw Motion"=FALSE) -> (w534:T15)
      n225 = shared-variable ".\\hatchPanelSharedVars.lvlib\\hatchPanelNotifier"() -> (w535:refnum<notifier>)  [unwired: 1 in, 1 out]
      n226 = shared-variable ".\\hatchPanelSharedVars.lvlib\\hatchPanelScored"() -> (w549:bool)  [unwired: 1 in, 1 out]
      n227 = Select(t=0.25, s=w541, f=w538) -> (s? t:f=w539:dbl)
      n228 = shared-variable ".\\driveSharedVars.lvlib\\driveMoveToTargetPower"(w539) -> ()  [unwired: 1 in, 1 out]
      n229 = shared-variable ".\\sonarSharedVars.lvlib\\sonarBrakeNotifier"() -> (w547:refnum<notifier>)  [unwired: 1 in, 1 out]
      n230 = Send Notification(notification=w534, notifier=w535) -> ()  [unwired: 1 in, 2 out]
      n231 = Select(t=AutoDriveStates."25 - Scored", s=w549, f=w548) -> (s? t:f=w526:T4)
      n232 = Send Notification(notification=TRUE, notifier=w547) -> ()  [unwired: 1 in, 2 out]
      n233 = shared-variable ".\\sensorsSharedVars.lvlib\\driveAvgVel(inch per s)"() -> (w537:dbl)  [unwired: 1 in, 1 out]
    }
    frame "25 - Scored" {
      n234 = Bundle By Name(cluster=T15 {"Hatch Panel State"=enum."Extended Closed", "Mechanism Motion"=FALSE, "Gathering Claw Motion"=FALSE, "Scoring Claw Motion"=FALSE} ("notification"), "Hatch Panel State"=hatchPanelEnum."Stach Mode", "Mechanism Motion"=FALSE, "Gathering Claw Motion"=FALSE, "Scoring Claw Motion"=FALSE) -> (w559:T15)
      n235 = shared-variable ".\\hatchPanelSharedVars.lvlib\\hatchPanelNotifier"() -> (w560:refnum<notifier>)  [unwired: 1 in, 1 out]
      n236 = shared-variable ".\\sonarSharedVars.lvlib\\sonarBrakeNotifier"() -> (w566:refnum<notifier>)  [unwired: 1 in, 1 out]
      n237 = Send Notification(notification=w559, notifier=w560) -> ()  [unwired: 1 in, 2 out]
      n238 = Send Notification(notification=FALSE, notifier=w566) -> ()  [unwired: 1 in, 2 out]
      n239 = shared-variable ".\\sensorsSharedVars.lvlib\\driveAvgVel(inch per s)"() -> (w562:dbl)  [unwired: 1 in, 1 out]
      n240 = Tick Count (ms)() -> (millisecond timer value=w563:u32)
    }
    frame "26 - Backup 0.3 Seconds" {
      n241 = Add(x=w577, y=u32 300) -> (x+y=w580:u32)
      n242 = shared-variable ".\\driveSharedVars.lvlib\\codeDriveThrottle"(-1.0 ("codeDriveThrottle")) -> ()  [unwired: 1 in, 1 out]
      n243 = shared-variable ".\\driveSharedVars.lvlib\\codeDriveSteer"(0.0 ("codeDriveSteer")) -> ()  [unwired: 1 in, 1 out]
      n244 = Tick Count (ms)() -> (millisecond timer value=w581:u32)
      n245 = Greater Or Equal?(x=w581, y=w580) -> (x >= y?=w579:bool)
      n246 = shared-variable ".\\sensorsSharedVars.lvlib\\driveAvgVel(inch per s)"() -> (w571:dbl)  [unwired: 1 in, 1 out]
      n247 = Select(t=AutoDriveStates."27 - doNothing", s=w579, f=w576) -> (s? t:f=w575:T4)
    }
    frame "27 - doNothing" {
      # "100"
      # "8.34457"
    }
  }
  "Drive State" <- w35
  n248 = feedback-in #1(w34) -> ()
  n249 = feedback-in #2(w8) -> ()
  n250 = feedback-in #3(w11) -> ()
  n251 = shared-variable ".\\hatchPanelSharedVars.lvlib\\hatchPanelReadyToScore"(w32) -> ()  [unwired: 1 in, 1 out]
  n252 = shared-variable ".\\limelightSharedVars.lvlib\\LimelightPipelineMode"(w3) -> ()  [unwired: 1 in, 1 out]
  n253 = case shown="\"High\"" w16 {
    tunnel: [TRUE FALSE] -> w15
    frame "Low", Default {
    }
    frame "High" {
    }
  }
  n254 = shared-variable ".\\TDMS.lvlib\\TDMS DevRef"() -> (w12:T19)  [unwired: 1 in, 1 out]
  n255 = shared-variable ".\\driveSharedVars.lvlib\\LowGear?"(w15) -> ()  [unwired: 1 in, 1 out]
  n256 = call <userlib>:"Logger_Log_Data.vi"("Data"=w11, "Channel"="Auto_Drive_State", "Group"="Robot_Data", "TDMS DevRef"=w12) -> ()  [unwired: 7 in, 1 out]
